vi "AuthMessage.vi"(8 "error in (no error)":errorcluster, 9 "Authenticate Extra  Data":T1, 10 "Challenge data":T2, 11 "WampScramAuthenticator in":refnum<class "WampScramAuthenticator.lvclass">) -> (0 "error out":errorcluster, 2 "AuthMessage":string, 3 "WampScramAuthenticator out":refnum<class "WampScramAuthenticator.lvclass">)   [LabVIEW 2020, in "wamplv.lvlib" / "WampScramAuthenticator.lvclass"]
uses:
  WampScramAuthenticator.lvclass
  TypeDefs/Challenge data.ctl
  TypeDefs/Authenticate Extra data.ctl
  WampScramAuthenticator.lvclass/WampScramAuthenticator.ctl
  TypeDefs/HMAC parameters.ctl
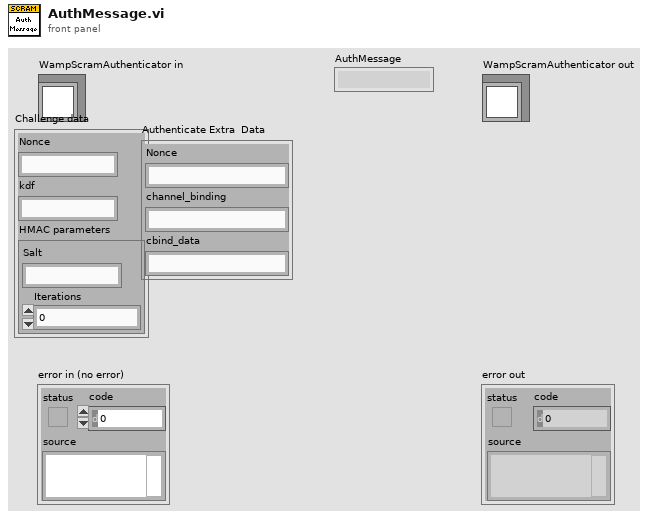
[diagram p1: front panel]
types:
  T1 = typedef "wamplv.lvlib/WampScramAuthenticator.lvclass/Authenticate Extra data.ctl" = cluster{"Nonce":string, "channel_binding":string, "cbind_data":string}
  T2 = typedef "wamplv.lvlib/WampScramAuthenticator.lvclass/Challenge data.ctl" = cluster{"Nonce":string, "kdf":string, "HMAC parameters":T3}
  T3 = typedef "wamplv.lvlib/WampScramAuthenticator.lvclass/HMAC parameters.ctl" = cluster{"Salt":string, "Iterations":i32}
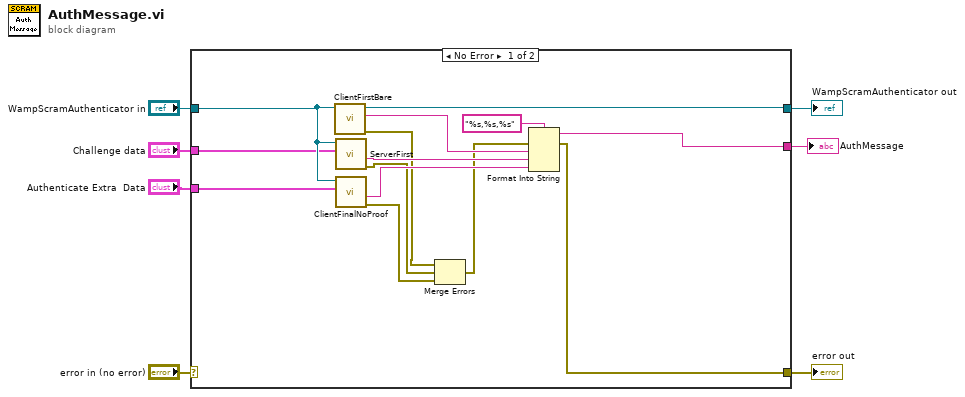
[diagram p0: block diagram]
diagram:
  n1 = case shown="No Error" "error in (no error)" {
    selector: "error in (no error)" -> [_ w23]
    tunnel: [w9 w23] -> w6
    tunnel: [w20 w22] -> w4
    tunnel: "WampScramAuthenticator in" -> [w21 w22]
    tunnel: "Challenge data" -> [w19 _]
    tunnel: "Authenticate Extra  Data" -> [w18 _]
    tunnel: [w8 _] -> w1
    frame No Error {
      n2 = call "ClientFirstBare.vi"("WampScramAuthenticator in"=w21) -> ("error out"=w13:errorcluster, "ClientFirstBare"=w16:string, "WampScramAuthenticator out"=w20:refnum<class "WampScramAuthenticator.lvclass">)  [unwired: 8 in]
      n3 = call "ServerFirst.vi"("Challenge data"=w19, "WampScramAuthenticator in"=w21) -> ("error out"=w12:errorcluster, "ServerFirst"=w15:string)  [unwired: 6 in, 2 out]
      n4 = call "ClientFinalNoProof.vi"("Authenticate Extra  Data"=w18, "WampScramAuthenticator in"=w21) -> ("error out"=w11:errorcluster, "ClientFinalNoProof"=w14:string)  [unwired: 6 in, 2 out]
      n5 = Merge Errors(w13, w12, w11) -> (w10:errorcluster)
      n6 = Format Into String(format string="%s,%s,%s", error in=w10, w16, w15, w14) -> (resulting string=w8:string, error out=w9:errorcluster)  [unwired: 1 in]
    }
    frame Error {
    }
  }
  "error out" <- w6
  "WampScramAuthenticator out" <- w4
  "AuthMessage" <- w1
